vi "Test Coffee Shop Removed Customer not Listed.vi"(8 "error in (no error)":errorcluster, 11 "Coffee Shop Test In":refnum<class "Coffee Shop Test.lvclass">) -> (0 "error out":errorcluster, 3 "Coffee Shop Test Out":refnum<class "Coffee Shop Test.lvclass">)   [LabVIEW 2020, in "Coffee Shop Test.lvclass"]
uses:
  Coffee Shop Test.lvclass
  C:/Program Files (x86)/National Instruments/LabVIEW 2020/vi.lib/Asteme/LUnit/Test Case.lvclass
  Coffee Shop/Coffee Shop.lvclass
  C:/Program Files (x86)/National Instruments/LabVIEW 2020/vi.lib/Asteme/Triarc Framework/Process/Process.lvclass
  <vilib>/Asteme/LUnit/Test Case.lvclass/Test Case.ctl
  <vilib>/Asteme/LUnit/LUnit Assertion Result.lvclass/LUnit Assertion Result.ctl
  <vilib>/Asteme/Triarc Framework/Process/Process.lvclass/Process.ctl
  <vilib>/Asteme/LUnit/Palette/Pass.vi
  <vilib>/Asteme/LUnit/Palette/Fail.vi
  <vilib>/Asteme/LUnit/Variant to string.vi
  <vilib>/Asteme/LUnit/Set Assertion Type.vi
  <vilib>/Asteme/Triarc Framework/Process/Private/SubVIs/Wait for finish.vi
  <vilib>/Asteme/Triarc Framework/Process/Protected/Messaging/Enqueue Message.vi
  <vilib>/Asteme/Triarc Framework/Process/Private/SubVIs/Set Lifecycle State.vi
  <vilib>/Asteme/Triarc Framework/Process/Public/Lifecycle/Get Lifecycle State.vi
  <vilib>/Asteme/LUnit/Add test result.vi
  <vilib>/Asteme/LUnit/LUnit Write Passed.vi
  <vilib>/Asteme/LUnit/LUnit Get Test Case.vi
  <vilib>/Asteme/LUnit/Assertion Result/LUnit Get Test Name.vi
  <vilib>/Asteme/LUnit/LUnit Write Message.vi
  <vilib>/Asteme/LUnit/LUnit Write Description.vi
  <vilib>/Asteme/LUnit/LUnit Write Assertion Type.vi
  <vilib>/Utility/error.llb/Clear Errors.vi
  <vilib>/Asteme/LUnit/Read Test Case Name.vi
  <vilib>/Utility/Data Type/Get Type Information.vi
  <vilib>/Utility/LVClass/Get LV Class Name.vi
  <vilib>/Utility/error.llb/Error Cluster From Error Code.vi
  <vilib>/Asteme/LUnit/LUnit Assertion Result.lvclass
  <vilib>/Asteme/Triarc Framework/Process/Process.lvclass
  <vilib>/Asteme/LUnit/Test Case.lvclass
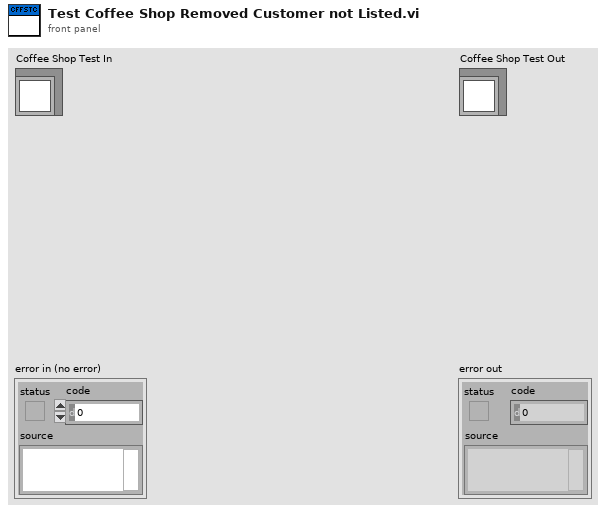
[diagram p1: front panel]
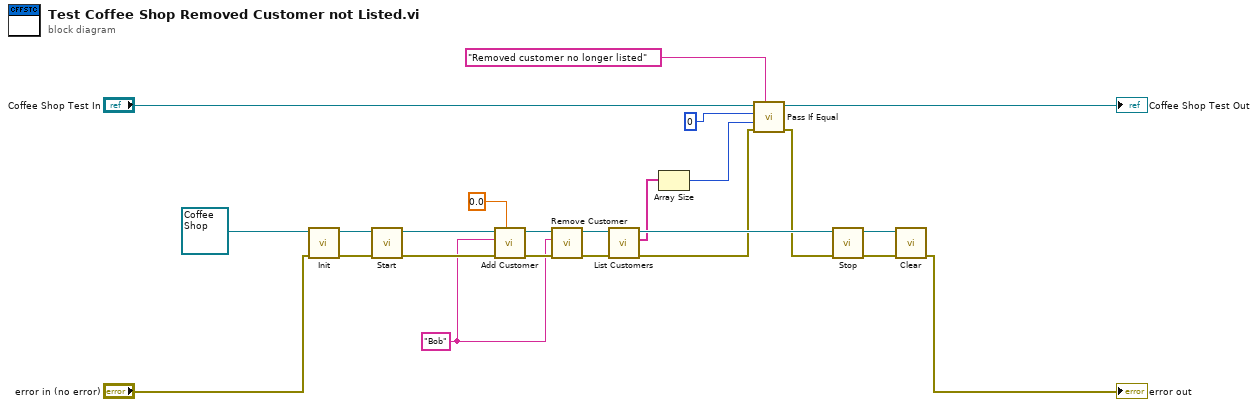
[diagram p0: block diagram]
diagram:
  w8 = "Bob" ("Name")
  n1 = call-dynamic "Init.vi"("error in (no error)"="error in (no error)", "Process In"=refnum<class "Coffee Shop.lvclass"> refnum ("Coffee Shop.lvclass")) -> ("error out"=w22:errorcluster, "Process Out"=w23:refnum<class "Coffee Shop.lvclass">)  [unwired: 8 in]
  n2 = call <vilib>:"Start.vi"("error in (no error)"=w22, "Process In"=w23) -> ("error out"=w17:errorcluster, "Process Out"=w16:refnum<class "Coffee Shop.lvclass">)  [unwired: 8 in]
  n3 = call "Add Customer.vi"("Delay Before Leaving [s]"=0.0, "error in (no error)"=w17, "Name"=w8, "Coffee Shop in"=w16) -> ("error out"=w18:errorcluster, "Coffee Shop out"=w10:refnum<class "Coffee Shop.lvclass">)  [unwired: 6 in]
  n4 = call "Remove Customer.vi"("error in (no error)"=w18, "Name"=w8, "Coffee Shop In"=w10) -> ("error out"=w11:errorcluster, "Coffee Shop Out"=w9:refnum<class "Coffee Shop.lvclass">)  [unwired: 7 in]
  n5 = call "List Customers.vi"("error in (no error)"=w11, "Coffee Shop in"=w9) -> ("error out"=w5:errorcluster, "Names"=w4:string[], "Coffee Shop out"=w12:refnum<class "Coffee Shop.lvclass">)  [unwired: 7 in]
  n6 = Array Size(array=w4) -> (size(s)=w2:i32)
  n7 = call <vilib>:"Pass If Equal.vi"("Description"="Removed customer no longer listed", "error in (no error)"=w5, "Actual"=w2, "Expected"=0 ("size(s)"), "Test Case In"="Coffee Shop Test In") -> ("error out"=w7:errorcluster, "Test Case Out"=→"Coffee Shop Test Out":refnum<class "Coffee Shop Test.lvclass">)  [unwired: 5 in]
  n8 = call <vilib>:"Stop.vi"("error in (no error)"=w7, "Process In"=w12) -> ("error out"=w20:errorcluster, "Process Out"=w21:refnum<class "Coffee Shop.lvclass">)  [unwired: 7 in, 1 out]
  n9 = call-dynamic "Clear.vi"("error in (no error)"=w20, "Application In"=w21) -> ("error out"=→"error out":errorcluster)  [unwired: 9 in]
